vi "Ephemeral RSA Testing.vi"() -> ()   [LabVIEW 2021]
uses:
  Key Management/CNG Key Info.ctl
  Key Management/CNG Provider Type.ctl
  Asymmetric Encryption/RSAEncryptionPadding.ctl
  Key Management/dotNET Crypto Key Management.lvlib
  Asymmetric Encryption/dotNET Crypto Asymmetric Encryption.lvlib
panel:
  out "error out":errorcluster
  out "encrypted data":string
  out "decrypted data":string
  out "Key Information":T1
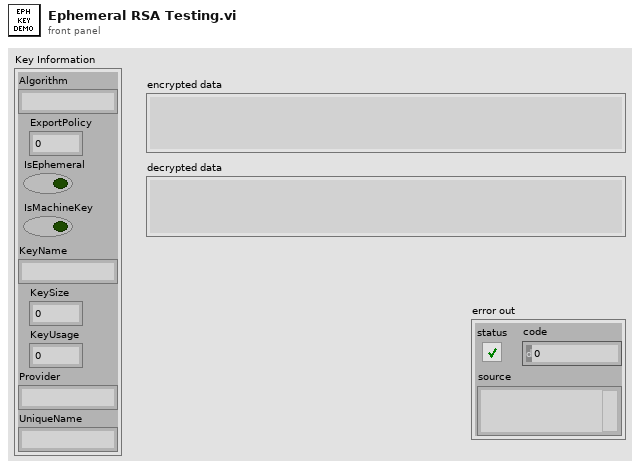
[diagram p1: front panel]
types:
  T1 = typedef "dotNET Crypto Key Management.lvlib/CNG Key Info.ctl" = cluster{"Algorithm":string, "ExportPolicy":i32, "IsEphemeral":bool, "IsMachineKey":bool, "KeyName":string, "KeySize":i32, "KeyUsage":i32, "Provider":string, "UniqueName":string}
  T2 = typedef "dotNET Crypto Asymmetric Encryption.lvlib/RSAEncryptionPadding.ctl" = enum16{"OaepSHA1", "OaepSHA256", "OaepSHA384", "OaepSHA512", "Pkcs1"}
  T3 = typedef "dotNET Crypto Key Management.lvlib/CNG Provider Type.ctl" = enum16{"Microsoft Software Key Storage Provider", "Microsoft Platform Crypto Provider"}
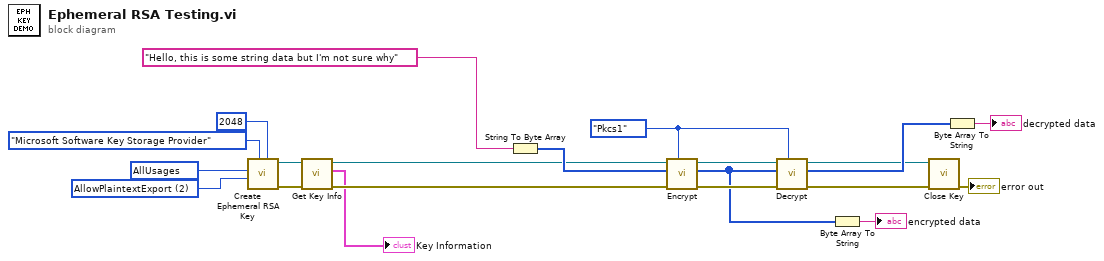
[diagram p0: block diagram]
diagram:
  w12 = RSAEncryptionPadding."Pkcs1" ("Padding Mode")
  w15 = 2 items=["None"=0, "AllowExport"=1, "AllowPlaintextExport"=2, "AllowArchiving"=4, "AllowPlaintextArchiving"=8] ("Export Policy (allow export)")
  w16 = 16777215 items=["None"=0, "Decryption"=1, "Signing"=2, "KeyAgreement"=4, "AllUsages"=16777215] ("Key Usage (all usages)")
  n1 = call "Create Ephemeral RSA Key.vi"("Key Length (2048)"=2048, "Crypto Provider"=CNG_Provider_Type."Microsoft Software Key Storage Provider", "Export Policy (allow export)"=w15, "Key Usage (all usages)"=w16) -> ("error out"=w20:errorcluster, "CngKey out"=w18:refnum<k24>)  [unwired: 6 in]
  n2 = call "Get Key Info.vi"("error in (no error)"=w20, "CngKey in"=w18) -> ("error out"=w19:errorcluster, "Key Information"=→"Key Information":T1, "CngKey out"=w1:refnum<k24>)  [unwired: 7 in]
  n3 = String To Byte Array(string="Hello, this is some string data but I'm not sure why") -> (unsigned byte array=w7:u8[])
  n4 = call "Encrypt.vi"("Padding Mode"=w12, "error in (no error)"=w19, "Raw data in"=w7, "CngKey in"=w1) -> ("error out"=w21:errorcluster, "Encrypted data out"=w3:u8[], "CngKey out"=w2:refnum<k24>)  [unwired: 5 in]
  n5 = call "Decrypt.vi"("Padding Mode"=w12, "error in (no error)"=w21, "Encrypted data in"=w3, "CngKey in"=w2) -> ("error out"=w6:errorcluster, "Raw data out"=w11:u8[], "CngKey out"=w5:refnum<k24>)  [unwired: 5 in]
  n6 = Byte Array To String(unsigned byte array=w3) -> (string=→"encrypted data":string)
  n7 = call "Close Key.vi"("error in (no error)"=w6, "CngKey in"=w5) -> ("error out"=→"error out":errorcluster)  [unwired: 9 in]
  n8 = Byte Array To String(unsigned byte array=w11) -> (string=→"decrypted data":string)
